vi "DAQ-Access-REv.vi"() -> ()   [LabVIEW 2024]
uses:
  <vilib>/DAQmx/read.llb/DAQmx Read (Analog 1D Wfm NChan NSamp).vi
  <vilib>/Analysis/baseanly.llb/Real A x B.vi
  <vilib>/Analysis/baseanly.llb/Mean (DBL).vi
  <vilib>/DAQmx/create/channels.llb/DAQmx Create Channel (AI-Voltage-Basic).vi
  <vilib>/DAQmx/configure/timing.llb/DAQmx Timing (Sample Clock).vi
  <vilib>/DAQmx/miscellaneous.llb/DAQmx Fill In Error Info.vi
  <vilib>/Waveform/WDTOps.llb/WDT Index Channel DBL.vi
  <vilib>/Analysis/Matrix/Numeric/Conversions/Matrix To Array - RM.vi
  <vilib>/Analysis/NI_AALBase.lvlib
  <vilib>/Analysis/Matrix/NI_Matrix.lvlib
panel:
  out "Force":waveform(dbl)[](graph)
  out "Raw AD":waveform(dbl)[](graph)
  out "Filename Out":path
  out "Data Writing":bool caption="Saving Data"
  out "Force Array (F)   -> Time":dbl[][](array[numeric]) format="%#.3f"
  in  "Convert Matrix":dbl[][](array[numeric])=[[0.01787384, 0.5614992, -0.6825333], [-0.80829626, 0.31005788, 0.3553213], [0.6880116, 0.4358145, 0.7359737]]
  in  "StopAll":bool
  out "How many time get offset":i32
  out "Ch3 Origin":dbl
  out "Ch2 Origin":dbl
  out "Ch1 Origin":dbl
  out "RawCantilever (V)\n (Offset removed     -> Time)":dbl[][](array[numeric]) format="%#.3f"
  out "C 3":dbl[](array[numeric]) format="%#.5g"
  out "C 2":dbl[](array[numeric]) format="%#.5g"
  out "C1":dbl[](array[numeric]) format="%#.5g"
  in  "Get Orogin":bool
  in  "samples per channel":i32=500
  in  "sample mode":i32(ring)=10123 items=["Continuous Samples"=10123, "Finite Samples"=10178, "Hardware Timed Single Point"=12522]
  in  "rate":dbl=1000.0 format="%0.2f"
  in  "physical channels":tag="Dev2/ai0:2"
  # "Connect USB6009 ch1,2,3 Analog Output on Amplifire unit\nConnect USB6009 ch1,2,3 =5V & GND on PowerIN on Amlofire unit"
  # "Phy Channel -> Set to 0-2\nRate 1000Hz\nSampleMode  -> Contenious Sampling\nSample per Channel -> 100"
  # "Device Setting"
  # "Main Graph"
  # "Zero Operation"
  # "Data File Writing"
  # "Support Information"
  # "Raw A/D (V)"
  # "C1"
  # "Shear X"
  # "C2"
  # "Shear Y"
  # "Offset (V)"
  # "C3"
  # "Force Z"
  # "No.509 \n[[ 0.01787384, 0.5614992 , -0.6825333 ],\n[-0.80829626, 0.31005788, 0.3553213 ],\n[ 0.6880116 , 0.4358145 , 0.7359737 ]"
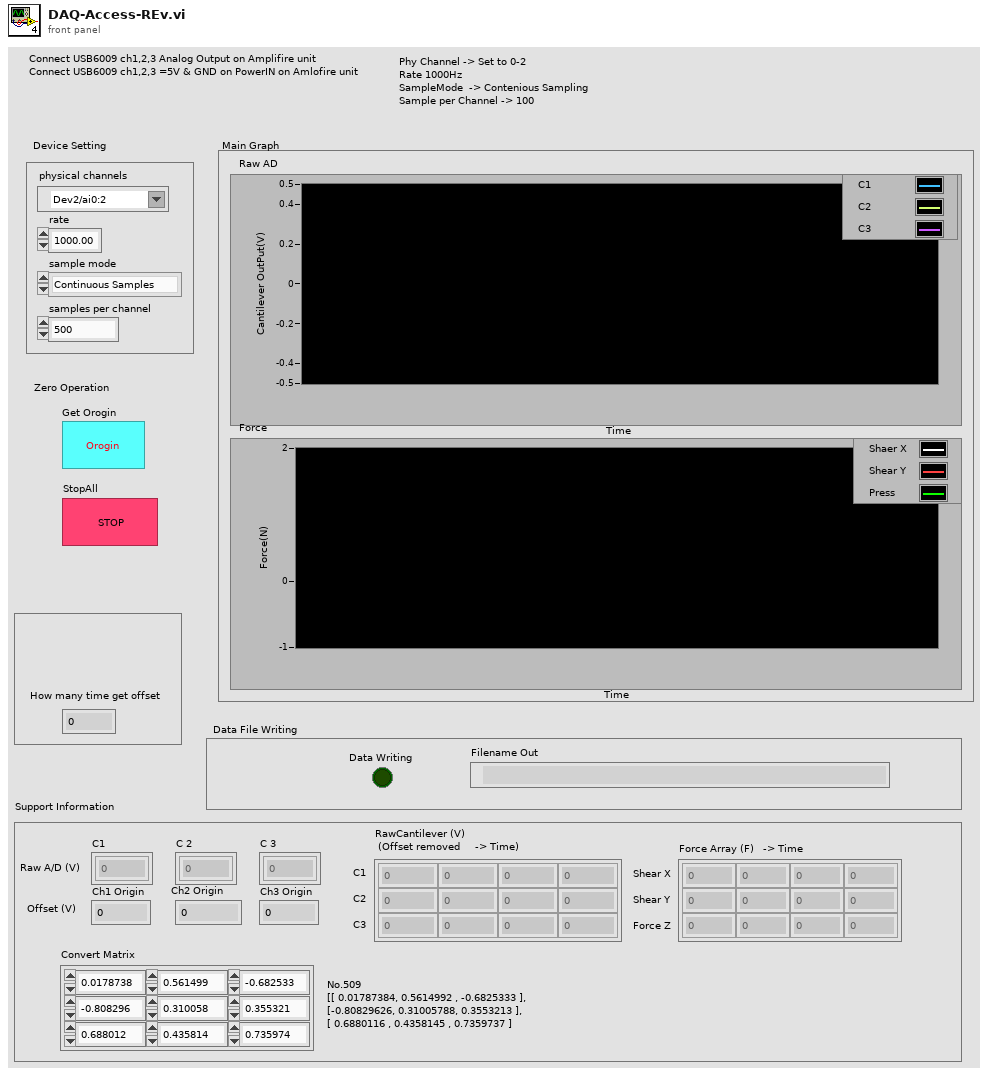
[diagram p1: front panel]
types:
  T1 = typedef "NI_Matrix.lvlib/RealMatrix.ctl" = dbl[][]
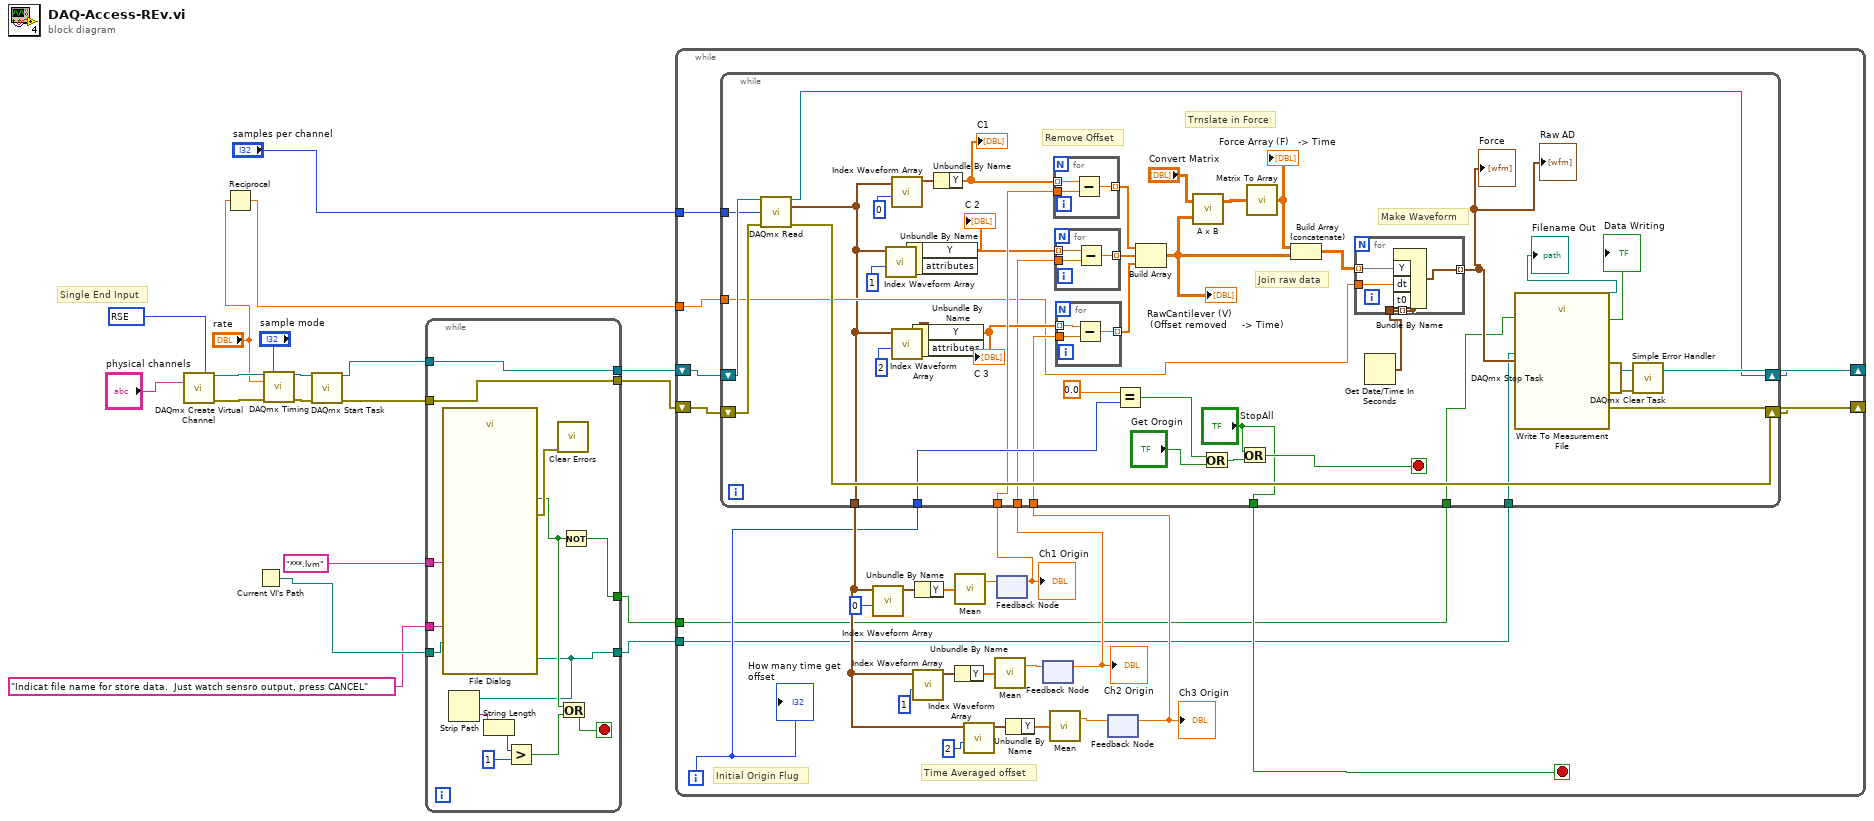
[diagram p0: block diagram]
diagram:
  w13 = 10083 items=["Default"=-1, "RSE"=10083, "NRSE"=10078, "Differential"=10106, "Pseudodifferential"=12529] ("input terminal configuration")
  # "Single End Input"
  n1 = call-poly <vilib>:"DAQmx Create Virtual Channel.vi"("input terminal configuration"=w13, "physical channels"="physical channels") -> ("task out"=w18:refnum<k21>, "error out"=w17:errorcluster)  [unwired: 12 in]
  n2 = Reciprocal(x="rate") -> (1/x=w10:dbl)
  n3 = Current VI's Path() -> (path=w4:path)
  n4 = call-poly <vilib>:"DAQmx Timing.vi"("task/channels in"=w18, "sample mode"="sample mode", "rate"="rate", "error in"=w17) -> ("task out"=w16:refnum<k21>, "error out"=w15:errorcluster)  [unwired: 10 in]
  n5 = call <vilib>:"DAQmx Start Task.vi"("task/channels in"=w16, "error in"=w15) -> ("task out"=w8:refnum<k21>, "error out"=w6:errorcluster)  [unwired: 12 in]
  n6 = while {
    tunnel: [w32] -> w1
    tunnel: [w37] -> w2
    tunnel: "Indicat file name for store data.  Just watch sensro output, press CANCEL" ("prompt") -> [w34]
    tunnel: "***.lvm" ("default name") -> [w28]
    tunnel: [w27] -> w9
    tunnel: w8 -> [w27]
    tunnel: [w26] -> w7
    tunnel: w6 -> [w26]
    tunnel: w4 -> [w25]
    stop <- w35 stop-if-true
    n7 = call "File Dialog"("start path"=w25, "prompt"=w34, "default name"=w28) -> ("selected path"=w32:path, "cancelled"=w36:bool, "error out"=w38:errorcluster)  [unwired: 9 in, 1 out]
    n8 = Strip Path(path=w32) -> (name=w33:string)  [unwired: 1 out]
    n9 = String Length(string=w33) -> (length=w31:i32)
    n10 = Greater?(x=w31, y=1) -> (0:w29:bool)
    n11 = call <vilib>:"Clear Errors.vi"("error in (no error)"=w38) -> ()  [unwired: 5 in, 2 out]
    n12 = Or(x=w36, y=w29) -> (x .or. y?=w35:bool)
    n13 = Not(x=w36) -> (.not. x?=w37:bool)
  }
  n14 = while {
    shift-right: [w61] -> w22
    shift-left: w9 -> [w64]
    shift-right: [w62] -> w23
    shift-left: w7 -> [w63]
    tunnel: w10 -> [w42]
    tunnel: "samples per channel" -> [w41]
    tunnel: w2 -> [w40]
    tunnel: w1 -> [w39]
    i -> [w52]
    stop <- w53 stop-if-true
    # "Time Averaged offset"
    # "Initial Origin Flug"
    n15 = feedback #1() -> (w48:dbl)  [unwired: 1 in]
    "Ch1 Origin" <- w48
    n16 = feedback #2() -> (w43:dbl)  [unwired: 1 in]
    "Ch2 Origin" <- w43
    n17 = feedback #3() -> (w44:dbl)  [unwired: 1 in]
    "Ch3 Origin" <- w44
    n18 = while {
      shift-right: [w101] -> w61
      shift-left: w64 -> [w104]
      shift-right: [w102] -> w62
      shift-left: w63 -> [w103]
      tunnel: [w71] -> w57
      tunnel: ["StopAll"] -> w53
      tunnel: w52 -> [w91]
      tunnel: w48 -> [w84]
      tunnel: w43 -> [w80]
      tunnel: w44 -> [w79]
      tunnel: w42 -> [w75]
      tunnel: w41 -> [w67]
      tunnel: w40 -> [w66]
      tunnel: w39 -> [w65]
      stop <- w94 stop-if-true
      # "Make Waveform"
      # "Trnslate in Force"
      # "Remove Offset"
      # "Join raw data"
      n19 = call-poly <vilib>:"DAQmx Read.vi"("task/channels in"=w104, "number of samples per channel"=w67, "error in"=w103) -> ("task out"=w101:refnum<k21>, "data"=w71:waveform(dbl)[], "error out"=w102:errorcluster)  [unwired: 10 in]
      n20 = call-poly <vilib>:"Index Waveform Array.vi"("index"=1, "waveform array"=w71) -> ("waveform"=w97:waveform(dbl))  [unwired: 8 in, 1 out]
      n21 = call-poly <vilib>:"Index Waveform Array.vi"("index"=0, "waveform array"=w71) -> ("waveform"=w99:waveform(dbl))  [unwired: 8 in, 1 out]
      n22 = call-poly <vilib>:"Index Waveform Array.vi"("index"=2, "waveform array"=w71) -> ("waveform"=w95:waveform(dbl))  [unwired: 8 in, 1 out]
      n23 = Unbundle By Name(w97) -> ("Y"=w82:dbl[])  [unwired: 1 out]
      "C 2" <- w82
      n24 = Unbundle By Name(w95) -> ("Y"=w81:dbl[])  [unwired: 1 out]
      "C 3" <- w81
      n25 = Unbundle By Name(w99) -> ("Y"=w85:dbl[])
      "C1" <- w85
      n26 = for {
        tunnel: w85 -> [w117] mode=indexing
        tunnel: w84 -> [w116]
        tunnel: [w115] -> w83 mode=indexing
        n27 = Subtract(x=w117, y=w116) -> (x-y=w115:dbl)
      }
      n28 = for {
        tunnel: [w114] -> w78 mode=indexing
        tunnel: w82 -> [w113] mode=indexing
        tunnel: w80 -> [w112]
        n29 = Subtract(x=w113, y=w112) -> (x-y=w114:dbl)
      }
      n30 = for {
        tunnel: [w111] -> w77 mode=indexing
        tunnel: w81 -> [w110] mode=indexing
        tunnel: w79 -> [w109]
        n31 = Subtract(x=w110, y=w109) -> (x-y=w111:dbl)
      }
      n32 = Equal?(x=0.0, y=w91) -> (x = y?=w90:bool)
      n33 = Build Array(w83, w78, w77) -> (w74:dbl[][])
      "RawCantilever (V)\n (Offset removed     -> Time)" <- w74
      n34 = call-poly <vilib>:"A x B.vi"("B"=w74, "A"="Convert Matrix") -> ("A x B"=w87:T1)  [unwired: 1 out]
      n35 = Or(x=w90, y="Get Orogin") -> (x .or. y?=w88:bool)
      n36 = Or(x="StopAll", y=w88) -> (x .or. y?=w94:bool)
      n37 = call-poly <vilib>:"Matrix To Array.vi"("Real Matrix"=w87) -> ("Real 2D Array"=w70:dbl[][])
      "Force Array (F)   -> Time" <- w70
      n38 = Build Array (concatenate)(w70, w74) -> (w73:dbl[][])
      n39 = Get Date/Time In Seconds() -> (seconds since 1Jan1904=w69:timestamp)
      n40 = for {
        tunnel: w73 -> [w106] mode=indexing
        tunnel: [w108] -> w68 mode=indexing
        tunnel: w75 -> [w107]
        tunnel: [w105] -> _ mode=indexing
        tunnel: w69 -> [w105]
        n41 = Bundle By Name("Y"=w106, "dt"=w107, "t0"=w105) -> (w108:waveform(dbl))  [unwired: 1 in]
      }
      "Raw AD" <- w68
      "Force" <- w68
      n42 = call "Write To Measurement File"("Signals"=w68, "Enable"=w66, "Filename"=w65) -> ("Filename Out"=→"Filename Out":path, "Saving Data"=→"Data Writing":bool)  [unwired: 14 in, 1 out]
    }
    n43 = call-poly <vilib>:"Index Waveform Array.vi"("index"=0, "waveform array"=w57) -> ("waveform"=w60:waveform(dbl))  [unwired: 8 in, 1 out]
    n44 = call-poly <vilib>:"Index Waveform Array.vi"("index"=1, "waveform array"=w57) -> ("waveform"=w59:waveform(dbl))  [unwired: 8 in, 1 out]
    n45 = Unbundle By Name(w60) -> ("Y"=w51:dbl[])
    n46 = call-poly <vilib>:"Mean.vi"("X"=w51) -> ("mean"=w49:dbl)  [unwired: 1 out]
    n47 = Unbundle By Name(w59) -> ("Y"=w50:dbl[])
    n48 = call-poly <vilib>:"Index Waveform Array.vi"("index"=2, "waveform array"=w57) -> ("waveform"=w58:waveform(dbl))  [unwired: 8 in, 1 out]
    n49 = call-poly <vilib>:"Mean.vi"("X"=w50) -> ("mean"=w47:dbl)  [unwired: 1 out]
    n50 = feedback-in #1(w49) -> ()
    n51 = Unbundle By Name(w58) -> ("Y"=w46:dbl[])
    n52 = feedback-in #2(w47) -> ()
    n53 = call-poly <vilib>:"Mean.vi"("X"=w46) -> ("mean"=w45:dbl)  [unwired: 1 out]
    n54 = feedback-in #3(w45) -> ()
    "How many time get offset" <- w52
  }
  n55 = call <vilib>:"DAQmx Stop Task.vi"("task/channels in"=w22, "error in"=w23) -> ("task out"=w20:refnum<k21>, "error out"=w21:errorcluster)  [unwired: 12 in]
  n56 = call <vilib>:"DAQmx Clear Task.vi"("task in"=w20, "error in"=w21) -> ("error out"=w19:errorcluster)  [unwired: 13 in]
  n57 = call <vilib>:"Simple Error Handler.vi"("error in (no error)"=w19) -> ()  [unwired: 4 in, 5 out]
